vi "MeasurementSelect.vi"() -> (0 "任务序号":i32[](array[numeric]))   [LabVIEW 2018]
uses:
  Selectable ListBox xControl/ListBox XControl.xctl
panel:
  out "Selected Items []":string[](array[string])
  in  "Get":bool
  in  "Invert":bool
  in  "Select None":bool
  in  "Select All":bool
  in  "任务选择":string[](xcontrol)
  # "选择要执行的测量任务后点击确定"
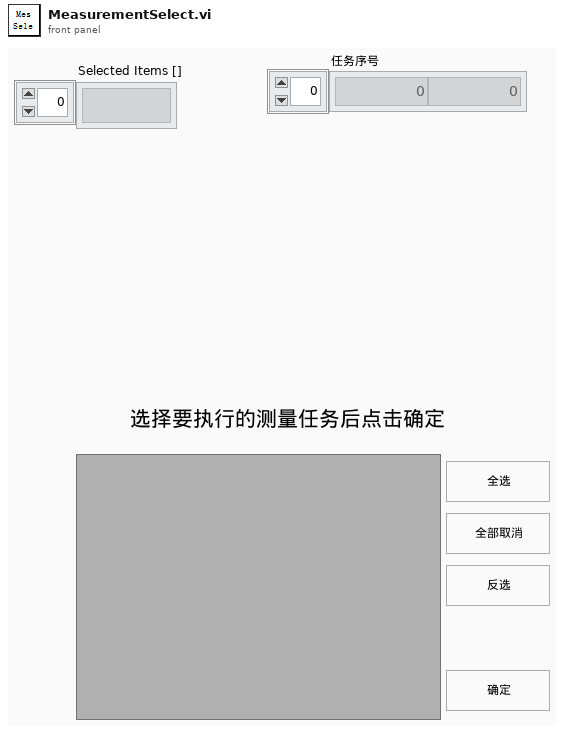
[diagram p1: front panel]
types:
  T1 = cluster{"Selected Index []":i32[], "Selected Items":string[], " 所有任务":string[], "任务布尔":bool[]}
  T2 = cluster{"任务":cluster{"功率任务":bool, "能量任务":bool, "时间波形任务":bool, "光谱任务":bool, "偏振任务":bool, "近远场任务":bool}, "通信":cluster{"功率通信":bool, "能量通信":bool, "时间波形通信":bool, "光谱通信":bool, "偏振通信":bool, "近远场通信":bool}}
  T3 = cluster{"Selected Index []":i32[], "Selected Items":string[], string[], bool[]}
  T4 = cluster{"功率任务":bool, "能量任务":bool, "时间波形任务":bool, "光谱任务":bool, "偏振任务":bool, "近远场任务":bool}
  T5 = cluster{"功率通信":bool, "能量通信":bool, "时间波形通信":bool, "光谱通信":bool, "偏振通信":bool, "近远场通信":bool}
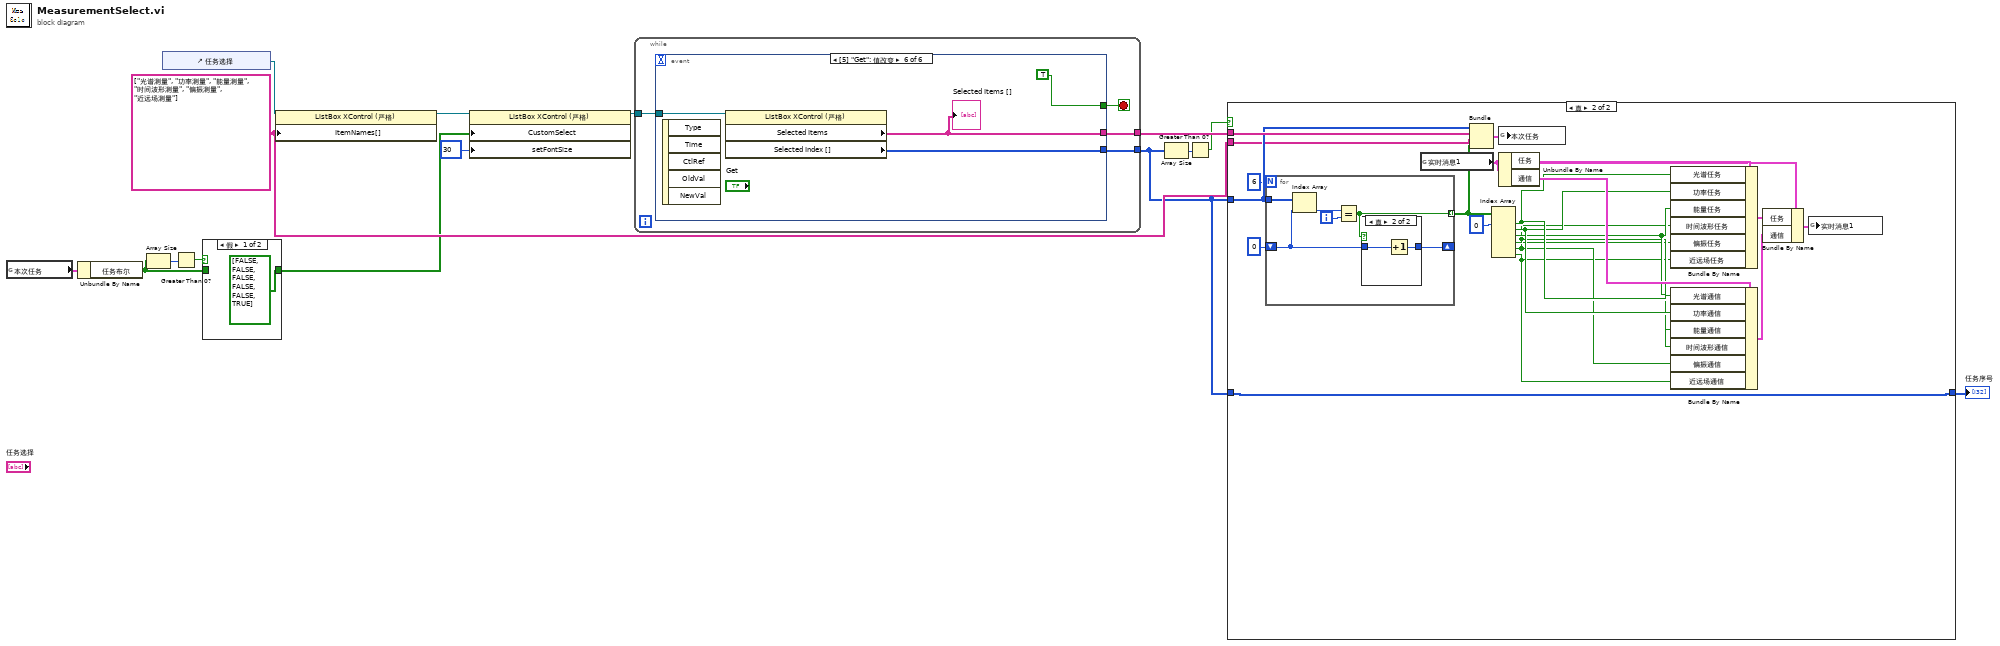
[diagram p0: block diagram]
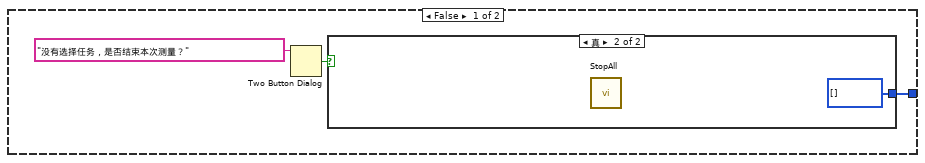
[diagram p2: hidden frame]
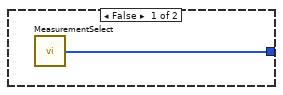
[diagram p3: hidden frame]
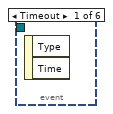
[diagram p5: hidden frame]
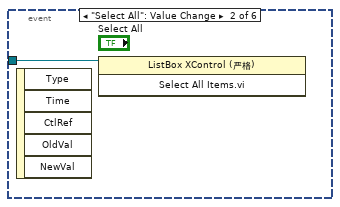
[diagram p6: hidden frame]
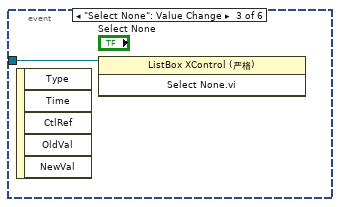
[diagram p7: hidden frame]
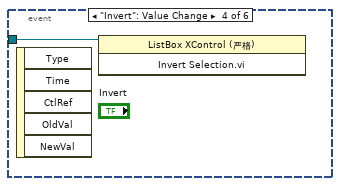
[diagram p8: hidden frame]
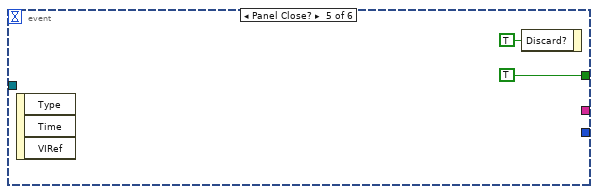
[diagram p9: hidden frame]
diagram:
  w12 = string[] ["光谱测量", "功率测量", "能量测量", "时间波形测量", "偏振测量", "近远场测量"]
  n1 = global read "参数.vi" "本次任务"() -> (w11:T1)
  n2 = Unbundle By Name(w11) -> ("任务布尔"=w8:bool[])
  n3 = Array Size(array=w8) -> (size(s)=w10:i32)
  n4 = control-ref of="任务选择"() -> (w14:refnum<vi>)
  n5 = Greater Than 0?(x=w10) -> (x > 0?=w9:bool)
  n6 = case shown="假" w9 {
    tunnel: w8 -> [_ w17]
    tunnel: [bool[] [FALSE, FALSE, FALSE, FALSE, FALSE, TRUE] ("任务布尔") w17] -> w7
    frame False {
    }
    frame True {
    }
  }
  n7 = property on="属性节点" class="ListBox XControl (严格)"(reference=w14, "ItemNames[]"=w12) -> (reference out=w13:refnum<vi>)  [unwired: 1 in, 1 out]
  n8 = property class="ListBox XControl (严格)"(reference=w13, "CustomSelect"=w7, "setFontSize"=u8 30) -> (reference out=w6:refnum<vi>)  [unwired: 1 in, 1 out]
  n9 = while {
    tunnel: w6 -> [w20]
    tunnel: [w19] -> w2
    tunnel: [w18] -> w15
    stop <- w21 stop-if-true
    n10 = event shown="[5] \"Get\": 值改变" {
      selector: _ -> [_ _ _ _ _ _]
      dyn-events: _ -> [_ _ _ _ _ _]
      timeout: _ -> [_ _ _ _ _ _]
      tunnel: [_ _ _ _ TRUE TRUE] -> w21
      tunnel: w20 -> [_ w22 w23 w24 _ w30]
      tunnel: [_ _ _ _ _ w28] -> w19
      tunnel: [_ _ _ _ _ w27] -> w18
      event Timeout {
        n11 = event-data() -> ()  [unwired: 1 in, 2 out]
      }
      event "Select All": Value Change {
        n12 = event-data() -> ()  [unwired: 1 in, 5 out]
        n13 = invoke on="调用节点" class="ListBox XControl (严格)" method="Select All Items.vi"(reference=w22) -> ()  [unwired: 2 in, 3 out]
      }
      event "Select None": Value Change {
        n14 = event-data() -> ()  [unwired: 1 in, 5 out]
        n15 = invoke on="调用节点" class="ListBox XControl (严格)" method="Select None.vi"(reference=w23) -> ()  [unwired: 2 in, 3 out]
      }
      event "Invert": Value Change {
        n16 = event-data() -> ()  [unwired: 1 in, 5 out]
        n17 = invoke on="调用节点" class="ListBox XControl (严格)" method="Invert Selection.vi"(reference=w24) -> ()  [unwired: 2 in, 3 out]
      }
      event Panel Close? {
        n18 = event-data() -> ()  [unwired: 1 in, 3 out]
        n19 = event-data("Discard?"=TRUE) -> ()  [unwired: 1 in, 1 out]
      }
      event "Get": Value Change {
        n20 = event-data() -> ()  [unwired: 1 in, 5 out]
        n21 = property on="属性节点" class="ListBox XControl (严格)"(reference=w30) -> ("Selected Items"=w27:string[], "Selected Index []"=w28:i32[])  [unwired: 1 in, 2 out]
        "Selected Items []" <- w27
      }
    }
  }
  n22 = Array Size(array=w2) -> (size(s)=w4:i32)
  n23 = Greater Than 0?(x=w4) -> (x > 0?=w3:bool)
  n24 = case shown="真" w3 {
    tunnel: w15 -> [_ w56]
    tunnel: w2 -> [_ w54]
    tunnel: w12 -> [_ w38]
    tunnel: w2 -> [_ w36]
    tunnel: [w31 w36] -> w1
    frame False {
      n25 = Two Button Dialog(message="没有选择任务，是否结束本次测量？" ("消息")) -> (T button?=w32:bool)  [unwired: 2 in]
      n26 = case shown="真" w32 {
        tunnel: [w34 i32[] [] ("任务序号")] -> w31
        frame False {
          n27 = call "MeasurementSelect.vi"() -> ("任务序号"=w34:i32[])  [unwired: 1 in]
        }
        frame True {
          n28 = call "StopAll.vi"() -> ()  [unwired: 12 in]
        }
      }
    }
    frame True {
      n29 = for {
        N: 6 -> [_]
        tunnel: w54 -> [w62]
        shift-right: [w58] -> _
        shift-left: 0 -> [w59]
        tunnel: [w57] -> w37 mode=indexing
        i -> [w60]
        n30 = Index Array(array=w62, index=w59) -> (element=w61:i32)
        n31 = Equal?(x=w61, y=w60) -> (x = y?=w57:bool)
        n32 = case shown="真" w57 {
          tunnel: w59 -> [w63 w65]
          tunnel: [w63 w64] -> w58
          frame False {
          }
          frame True {
            n33 = Increment(x=w65) -> (x+1=w64:i32)
          }
        }
      }
      n34 = global read "globalMessage.vi" "实时消息1"() -> (w49:T2)
      n35 = Bundle("Selected Index []"=w54, "Selected Items"=w56, w38, w37) -> (w55:T3)  [unwired: 1 in]
      n36 = Index Array(array=w37, index #1=0 ("索引")) -> (element #1=w45:bool, element #2=w44:bool, element #3=w43:bool, element #4=w42:bool, element #5=w41:bool, element #6=w40:bool)  [unwired: 5 in]
      n37 = global write "参数.vi" "本次任务"(w55) -> ()
      n38 = Unbundle By Name(w49) -> ("任务"=w50:T4, "通信"=w46:T5)
      n39 = Bundle By Name(cluster=w50, "光谱任务"=w45, "功率任务"=w44, "能量任务"=w43, "时间波形任务"=w42, "偏振任务"=w41, "近远场任务"=w40) -> (w47:T4)
      n40 = Bundle By Name(cluster=w46, "光谱通信"=w45, "功率通信"=w44, "能量通信"=w43, "时间波形通信"=w42, "偏振通信"=w41, "近远场通信"=w40) -> (w39:T5)
      n41 = Bundle By Name(cluster=w49, "任务"=w47, "通信"=w39) -> (w48:T2)
      n42 = global write "globalMessage.vi" "实时消息1"(w48) -> ()
    }
  }
  "任务序号" <- w1
